vi "run_file.vi"(8 "error in (no error)":errorcluster, 11 "filepath":path) -> (0 "error out":errorcluster)   [LabVIEW 2015, in "lv-bin-windows.lvlib" / "v1.lvlib"]
uses:
  v1.lvlib
  <vilib>/Utility/error.llb/Error Cluster From Error Code.vi
  <vilib>/ErrorRing/Error Ring.xnode
  <userlib>/antonio-alexander/lv-bin/lv-bin/public/api/v1/v1.lvlib
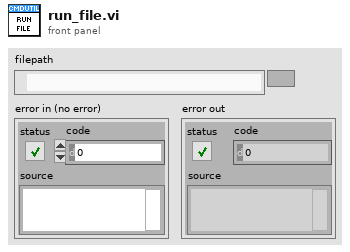
[diagram p1: front panel]
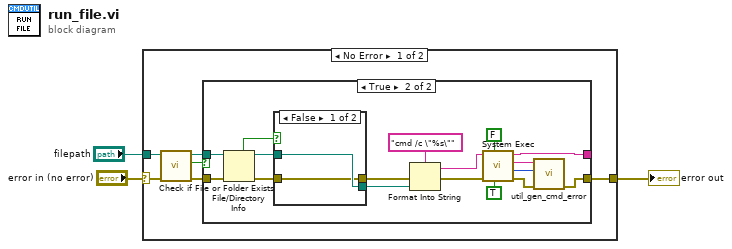
[diagram p0: block diagram]
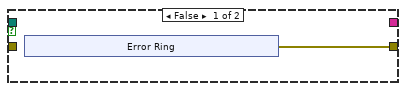
[diagram p2: hidden frame]
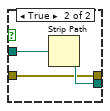
[diagram p3: hidden frame]
diagram:
  n1 = case shown="No Error" "error in (no error)" {
    selector: "error in (no error)" -> [w8 w37]
    tunnel: "filepath" -> [w6 _]
    tunnel: [w9 w37] -> w1
    frame No Error {
      n2 = call <vilib>:"Check if File or Folder Exists.vi"("error in (no error)"=w8, "path"=w6) -> ("error out"=w7:errorcluster, "file or folder exists?"=w4:bool, "dup path"=w5:path)  [unwired: 7 in]
      n3 = case shown="True" w4 {
        tunnel: w7 -> [_ w23]
        tunnel: w5 -> [_ w22]
        tunnel: [w10 w24] -> w9
        tunnel: [_ w27] -> _
        frame False {
          n4 = xnode "Error Ring"() -> ("error out"=w10:errorcluster)
        }
        frame True {
          n5 = File/Directory Info(path=w22, error in=w23) -> (path out=w20:path, directory=w21:bool, error out=w17:errorcluster)  [unwired: 4 out]
          n6 = case shown="False" w21 {
            tunnel: w20 -> [w33 w36]
            tunnel: [w33 w35] -> w19
            tunnel: [w32 w34] -> w18
            tunnel: w17 -> [w32 w34]
            frame False {
            }
            frame True {
              n7 = Strip Path(path=w36) -> (stripped path=w35:path)  [unwired: 1 out]
            }
          }
          n8 = Format Into String(format string="cmd /c \"%s\"", error in=w18, w19) -> (resulting string=w29:string, error out=w31:errorcluster)  [unwired: 1 in]
          n9 = call <vilib>:"System Exec.vi"("run minimized? (F)"=TRUE, "wait until completion? (T)"=FALSE, "error in (no error)"=w31, "command line"=w29) -> ("error out"=w25:errorcluster, "return code"=w15:i32, "standard error"=w16:string, "standard output"=w27:string)  [unwired: 4 in]
          n10 = call <userlib>:"util_gen_cmd_error.vi"("error in (no error)"=w25, "return_code"=w15, "standard_error"=w16) -> ("error out"=w24:errorcluster)  [unwired: 8 in]
        }
      }
    }
    frame Error {
    }
  }
  "error out" <- w1
